vi "buzzerTest.vi"() -> ()   [LabVIEW 2017]
panel:
  in  "Duty Cycle (0-1)":dbl
  in  "frequency [Hz]":dbl(slide) scale=0.0..40000.0
  in  "Stop Button":bool
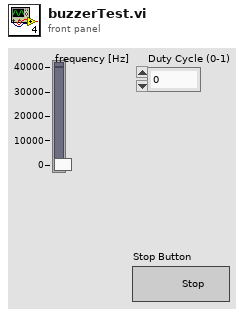
[diagram p1: front panel]
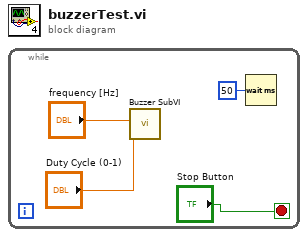
[diagram p0: block diagram]
diagram:
  n1 = while {
    stop <- "Stop Button" stop-if-true
    n2 = call "Buzzer SubVI.vi"("frequency [Hz]"="frequency [Hz]", "Duty Cycle (0-1)"="Duty Cycle (0-1)") -> ()  [unwired: 10 in]
    n3 = Wait (ms)(milliseconds to wait=u32 50) -> ()  [unwired: 1 out]
  }
